vi "SI_units_to_units_converter.vi"(2 "var_value in":dbl, 3 "String in":string) -> (0 "var_value out":dbl, 1 "String out":string)   [LabVIEW 2020]
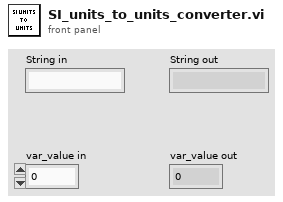
[diagram p1: front panel]
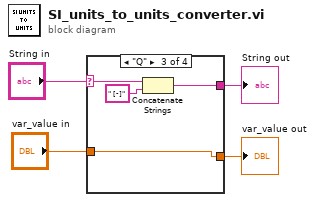
[diagram p0: block diagram]
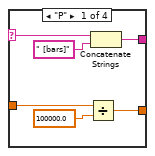
[diagram p2: hidden frame]
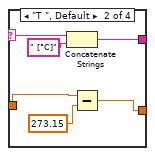
[diagram p3: hidden frame]
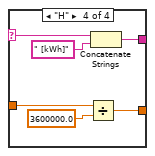
[diagram p4: hidden frame]
diagram:
  n1 = case shown="\"Q\"" "String in" {
    selector: "String in" -> [w7 w14 w19 w23]
    tunnel: [w10 w16 w20 w22] -> w1
    tunnel: "var_value in" -> [w8 w12 w20 w24]
    tunnel: [w5 w13 w17 w21] -> w3
    frame "P" {
      n2 = Divide(x=w8, y=100000.0) -> (x/y=w10:dbl)
      n3 = Concatenate Strings(w7, " [bars]") -> (w5:string)
    }
    frame "T ", Default {
      n4 = Concatenate Strings(w14, " [°C]") -> (w13:string)
      n5 = Subtract(x=w12, y=273.15) -> (x-y=w16:dbl)
    }
    frame "Q" {
      n6 = Concatenate Strings(w19, " [-]") -> (w17:string)
    }
    frame "H" {
      n7 = Divide(x=w24, y=3600000.0) -> (x/y=w22:dbl)
      n8 = Concatenate Strings(w23, " [kWh]") -> (w21:string)
    }
  }
  "String out" <- w3
  "var_value out" <- w1
